vi "sin_plot.vi"() -> ()   [LabVIEW 2014]
panel:
  in  "milliseconds to wait":u32=30 min=30
  in  "scale to ms":dbl=0.001 format="%#_13g"
  out "sin(x)":dbl(graph)
  out "iteration":dbl
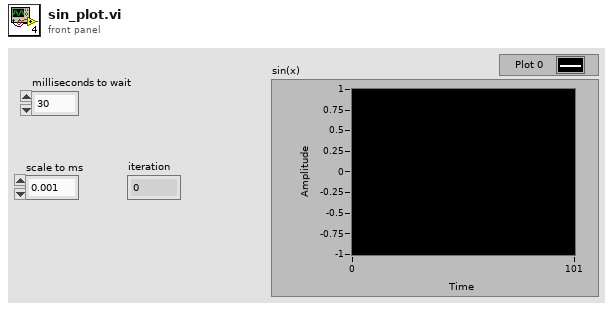
[diagram p1: front panel]
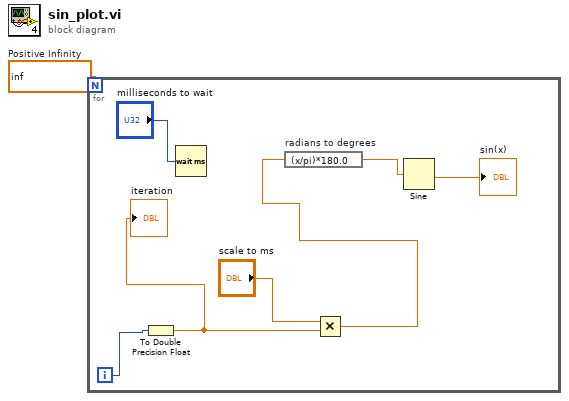
[diagram p0: block diagram]
diagram:
  w1 = inf  # Positive Infinity
  n1 = for {
    N: w1 -> [_]
    i -> [w6]
    n2 = To Double Precision Float(number=w6) -> (double precision float=w5:dbl)
    "iteration" <- w5
    n3 = Wait (ms)(milliseconds to wait="milliseconds to wait") -> ()  [unwired: 1 out]
    n4 = Multiply(x="scale to ms", y=w5) -> (x*y=w2:dbl)
    n5 = expression code="(x/pi)*180.0" "radians to degrees"(w2) -> (w3:dbl)
    n6 = Sine(x=w3) -> (sin(x)=→"sin(x)":dbl)
  }
